vi "CO Channel Config.vi"(8 "error in (no error)":errorcluster, 11 "Node Ptr":T2 format="%.0x") -> (0 "error out":errorcluster)   [LabVIEW 2011, in "Simulated Thermocouple Custom Device.lvlib"]
uses:
  Simulated Thermocouple Custom Device.lvlib
  <vilib>/NI Veristand/Custom Device API/Custom Device Item Ref.ctl
  <vilib>/NI Veristand/Custom Device API/Get Item Property (Variant).vi
  <vilib>/NI Veristand/Custom Device API/Get Item Property (String).vi
  <vilib>/NI Veristand/Custom Device API/Set Item Property (Variant).vi
  <vilib>/NI Veristand/Custom Device API/Set Item Property (String).vi
  <vilib>/regexp/Match Regular Expression.xnode
  <vilib>/NI Veristand/Custom Device API/Custom Device API.lvlib
panel:
  in  "Units":string="A"
  out "Address":string
  in  "Physical Channel":u16(ring) items=["0", "1", "2", "3", "4", "5", "6", "7", "8", "9", "10", "11", "12", "13", "14", "15", "16", "17", "18", "19", "20", "21", "22", "23", "24", "25", "26", "27", "28", "29", "30", "31"]
  in  "Header 3":cluster{"Section Name":string}={"Section Name"="Physical Channel"}
  in  "CO Channel Config":T1={"Initial Value"=0.0, "Range Min"=0.0, "Range Max"=0.02} {"Range Max" min=0.0 max=0.02 step=0.001; "Range Min" min=0.0 max=0.02 step=0.001}
  in  "Header 2":cluster{"Section Name":string}={"Section Name"="Current Channel Settings"}
  in  "Header":cluster{"Section Name":string}={"Section Name"="Current Channel Specifications"}
  in  "Description":string="This page allows you to modify the settings for the physical channel listed at the bottom of this page.  Use the Physical Channel selector to change the hardware resource associated with this Veristand channel."
  in  "Name":string
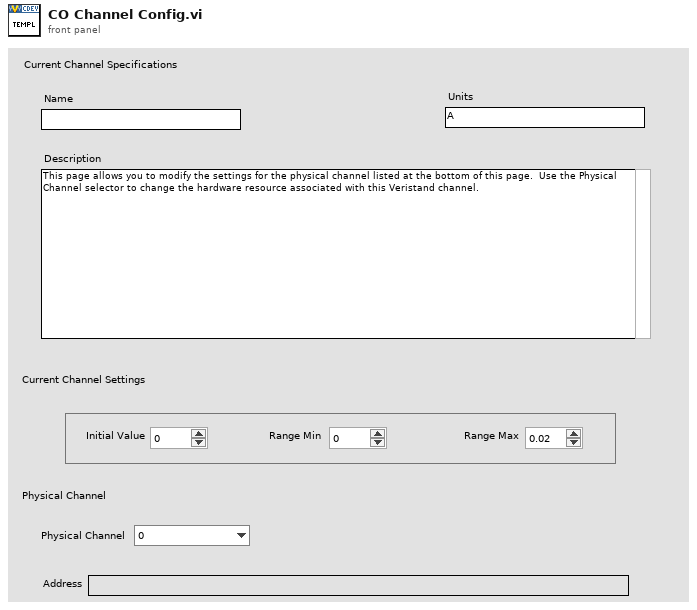
[diagram p1: front panel]
types:
  T1 = cluster{"Initial Value":dbl, "Range Min":dbl, "Range Max":dbl}
  T2 = typedef "Custom Device API.lvlib/Custom Device Item Ref.ctl" = u64
  T3 = typedef "Custom Device API.lvlib/Custom Device Item Info.ctl" = cluster{"Name":string, "Is Channel":bool, "GUID":string}
  T4 = typedef "Custom Device API.lvlib/Custom Device Commands.ctl" = enum16{"Default", "Item renamed", "Shutdown", "Dynamic button pressed"}
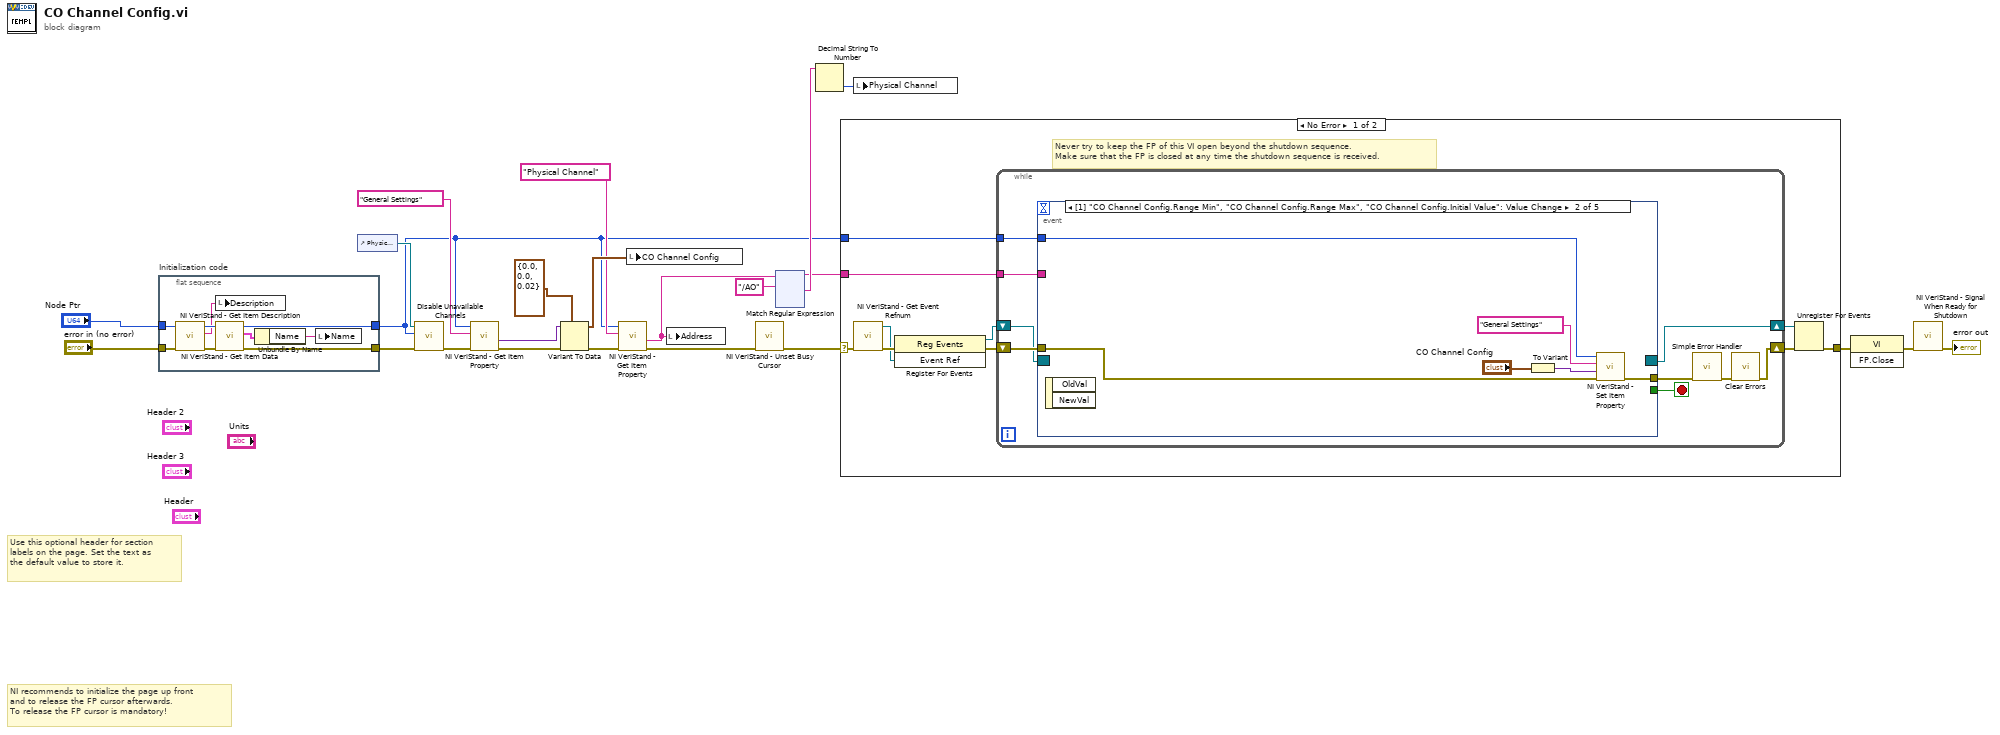
[diagram p0: block diagram]
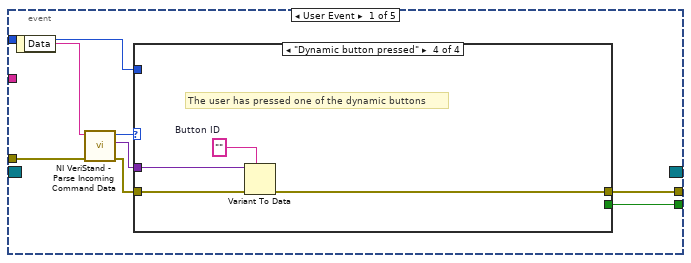
[diagram p2: hidden frame]
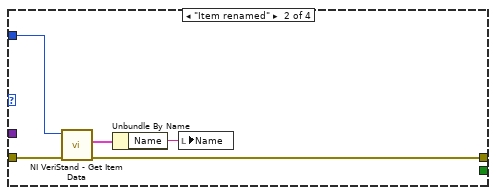
[diagram p4: hidden frame]
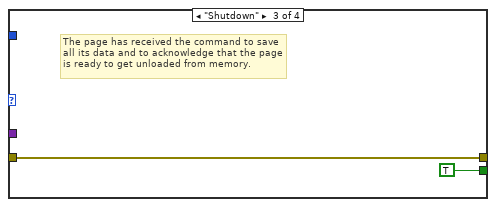
[diagram p5: hidden frame]
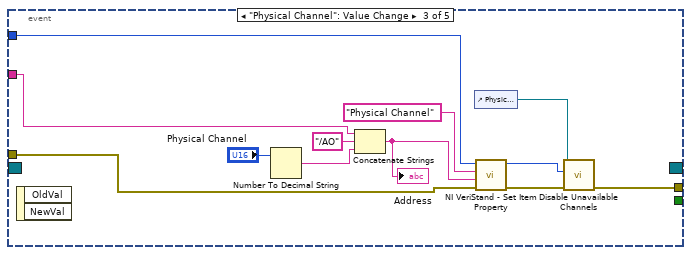
[diagram p6: hidden frame]
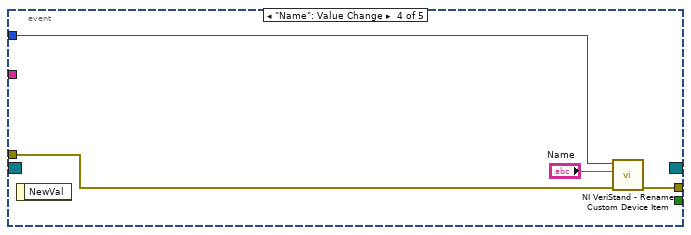
[diagram p7: hidden frame]
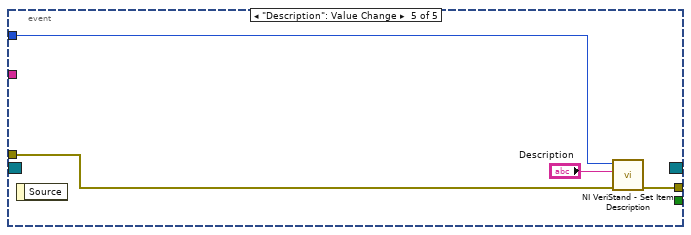
[diagram p8: hidden frame]
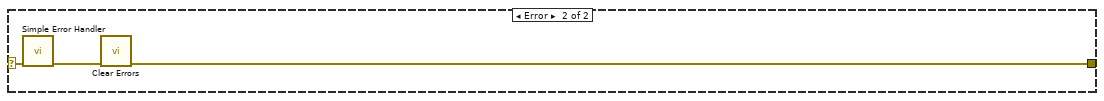
[diagram p9: hidden frame]
diagram:
  # "Use this optional header for section labels on the page. Set the text as the default value to store it."
  # "NI recommends to initialize the page up front\nand to release the FP cursor afterwards.\nTo release the FP cursor is mandatory!"
  n1 = flat-sequence "Initialization code" {
    tunnel: "error in (no error)" -> [w30]
    tunnel: "Node Ptr" -> [w29]
    tunnel: [w24] -> w17
    tunnel: [w32] -> w4
    frame #0 {
      n2 = call <vilib>:"NI VeriStand - Get Item Description.vi"("error in (no error)"=w30, "Item Ref in"=w29) -> ("error out"=w27:errorcluster, "Description"=w28:string, "Item Ref out"=w31:T2)  [unwired: 7 out]
      n3 = local write "Description"(w28) -> ()
      n4 = call <vilib>:"NI VeriStand - Get Item Data.vi"("error in (no error)"=w27, "Item Ref in"=w31) -> ("error out"=w24:errorcluster, "Item Info"=w26:T3, "Item Ref out"=w32:T2)  [unwired: 7 out]
      n5 = Unbundle By Name(w26) -> ("Name"=w25:string)
      n6 = local write "Name"(w25) -> ()
    }
  }
  n7 = control-ref of="Physical Channel"() -> (w16:refnum<vi>)
  n8 = call "Disable Unavailable Channels.vi"("error in (no error)"=w17, "Item Ref out"=w4, "Ring in"=w16) -> ("error out"=w15:errorcluster)  [unwired: 8 in]
  n9 = call-poly <vilib>:"NI VeriStand - Get Item Property.vi"("error in (no error)"=w15, "Property Name"="General Settings", "Item Ref in"=w4) -> ("error out"=w2:errorcluster, "Value"=w3:variant)  [unwired: 5 in, 2 out]
  n10 = Variant To Data(error in=w2, type=T1 {"Initial Value"=0.0, "Range Min"=0.0, "Range Max"=0.02} ("CO Channel Config"), Variant=w3) -> (data=w13:T1, error out=w12:errorcluster)
  n11 = call-poly <vilib>:"NI VeriStand - Get Item Property.vi"("error in (no error)"=w12, "Property Name"="Physical Channel", "Item Ref in"=w4) -> ("error out"=w7:errorcluster, "Value"=w11:string)  [unwired: 5 in, 2 out]
  n12 = local write "CO Channel Config"(w13) -> ()
  n13 = local write "Address"(w11) -> ()
  n14 = call <vilib>:"NI VeriStand - Unset Busy Cursor.vi"("error in (no error)"=w7) -> ("error out"=w19:errorcluster)  [unwired: 10 out]
  n15 = xnode "Match Regular Expression"("input string"=w11, "regular expression"="/AO") -> ("before match"=w6:string, "after match"=w9:string)  [unwired: 4 in, 3 out]
  n16 = Decimal String To Number(string=w9) -> (number=w8:i32)  [unwired: 2 in, 1 out]
  n17 = case shown="No Error" w19 {
    selector: w19 -> [w34 w100]
    tunnel: [w39 w98] -> w23
    tunnel: w4 -> [w35 _]
    tunnel: w6 -> [w33 _]
    frame No Error {
      # "Never try to keep the FP of this VI open beyond the shutdown sequence.\nMake sure that the FP is closed at any time the shutdown sequence is received."
      n18 = call <vilib>:"NI VeriStand - Get Event Refnum.vi"("error in (no error)"=w34) -> ("error out"=w42:errorcluster, "Event Ref"=w38:refnum<user-event>)  [unwired: 9 out]
      n19 = register-events(error in=w42, w38) -> (reference out=w36:refnum<event-registration>, error out=w37:errorcluster)  [unwired: 1 in]
      n20 = while {
        tunnel: w35 -> [w47]
        shift-right: [w44] -> w40
        shift-left: w37 -> [w50]
        shift-right: [w51] -> w41
        shift-left: w36 -> [w49]
        tunnel: w33 -> [w43]
        stop <- w48 stop-if-true
        n21 = event shown="[1] \"CO Channel Config.Range Min\", \"CO Channel Config.Range Max\", \"CO Channel Config.Initial Value\": Value Change" {
          selector: w49 -> [_ _ _ _ _]
          dyn-events: [_ _ _ _ _] -> w51
          timeout: _ -> [_ _ _ _ _]
          tunnel: w50 -> [w59 w73 w83 w93 w96]
          tunnel: [w55 _ _ _ _] -> w48
          tunnel: [w54 w72 w78 w92 w95] -> w46
          tunnel: w47 -> [w53 w75 w89 w91 w97]
          tunnel: w43 -> [_ _ w87 _ _]
          event User Event {
            n22 = event-data() -> ("Data"=w58:string)  [unwired: 1 out]
            n23 = call <vilib>:"NI VeriStand - Parse Incoming Command Data.vi"("error in (no error)"=w59, "Incoming data"=w58) -> ("error out"=w57:errorcluster, "Outgoing data"=w52:variant, "Action"=w56:T4)  [unwired: 7 out]
            n24 = case shown="\"Dynamic button pressed\"" w56 {
              tunnel: w57 -> [w60 w65 w66 w71]
              tunnel: [_ _ TRUE _] -> w55
              tunnel: [w60 w62 w66 w68] -> w54
              tunnel: w53 -> [_ w64 _ _]
              tunnel: w52 -> [_ _ _ w70]
              frame "Default", Default {
              }
              frame "Item renamed" {
                n25 = call <vilib>:"NI VeriStand - Get Item Data.vi"("error in (no error)"=w65, "Item Ref in"=w64) -> ("error out"=w62:errorcluster, "Item Info"=w63:T3)  [unwired: 8 out]
                n26 = Unbundle By Name(w63) -> ("Name"=w61:string)
                n27 = local write "Name"(w61) -> ()
              }
              frame "Shutdown" {
                # "The page has received the command to save all its data and to acknowledge that the page is ready to get unloaded from memory."
              }
              frame "Dynamic button pressed" {
                w69 = ""  # Button ID
                # "The user has pressed one of the dynamic buttons"
                n28 = Variant To Data(error in=w71, type=w69, Variant=w70) -> (error out=w68:errorcluster)  [unwired: 1 out]
              }
            }
          }
          event "CO Channel Config.Range Min", "CO Channel Config.Range Max", "CO Channel Config.Initial Value": Value Change {
            n29 = event-data() -> ()  [unwired: 3 out]
            n30 = To Variant(anything="CO Channel Config") -> (Variant=w76:variant)
            n31 = call-poly <vilib>:"NI VeriStand - Set Item Property.vi"("error in (no error)"=w73, "Value"=w76, "Property Name"="General Settings", "Item Ref in"=w75) -> ("error out"=w72:errorcluster)  [unwired: 5 in, 2 out]
          }
          event "Physical Channel": Value Change {
            n32 = event-data() -> ()  [unwired: 3 out]
            n33 = Number To Decimal String(number="Physical Channel") -> (decimal integer string=w85:string)  [unwired: 1 in]
            n34 = Concatenate Strings(w87, "/AO" ("regular expression"), w85) -> (w82:string)
            "Address" <- w82
            n35 = control-ref of="Physical Channel"() -> (w80:refnum<vi>)
            n36 = call-poly <vilib>:"NI VeriStand - Set Item Property.vi"("error in (no error)"=w83, "Value"=w82, "Property Name"="Physical Channel", "Item Ref in"=w89) -> ("error out"=w79:errorcluster, "Item Ref out"=w81:T2)  [unwired: 5 in, 1 out]
            n37 = call "Disable Unavailable Channels.vi"("error in (no error)"=w79, "Item Ref out"=w81, "Ring in"=w80) -> ("error out"=w78:errorcluster)  [unwired: 8 in]
          }
          event "Name": Value Change {
            n38 = event-data() -> ()  [unwired: 2 out]
            n39 = call <vilib>:"NI VeriStand - Rename Custom Device Item.vi"("error in (no error)"=w93, "New Name"="Name", "Item Ref in"=w91) -> ("error out"=w92:errorcluster)  [unwired: 8 out]
          }
          event "Description": Value Change {
            n40 = event-data() -> ()  [unwired: 2 out]
            n41 = call <vilib>:"NI VeriStand - Set Item Description.vi"("error in (no error)"=w96, "Description"="Description", "Item Ref in"=w97) -> ("error out"=w95:errorcluster)  [unwired: 8 out]
          }
        }
        n42 = call <vilib>:"Simple Error Handler.vi"("error in (no error)"=w46) -> ("error out"=w45:errorcluster)  [unwired: 1 in, 7 out]
        n43 = call <vilib>:"Clear Errors.vi"("error in (no error)"=w45) -> ("error out"=w44:errorcluster)  [unwired: 6 out]
      }
      n44 = Unregister For Events(event registration refnum=w41, error in=w40) -> (error out=w39:errorcluster)
    }
    frame Error {
      n45 = call <vilib>:"Simple Error Handler.vi"("error in (no error)"=w100) -> ("error out"=w99:errorcluster)  [unwired: 1 in, 7 out]
      n46 = call <vilib>:"Clear Errors.vi"("error in (no error)"=w99) -> ("error out"=w98:errorcluster)  [unwired: 6 out]
    }
  }
  n47 = local write "Physical Channel"(w8) -> ()
  n48 = invoke class="VI" method="FP.Close"(error in=w23) -> (error out=w22:errorcluster)  [unwired: 2 in, 2 out]
  n49 = call <vilib>:"NI VeriStand - Signal When Ready for Shutdown.vi"("error in (no error)"=w22) -> ("error out"=→"error out":errorcluster)  [unwired: 10 out]
